vi "dare_verify.vi"(7 "Answer":T1, 8 "Q":T1, 9 "R":T1, 10 "B":T1, 11 "A":T1) -> (0 "Eigenvalues":cdb[](array[numeric]), 1 "ZERO":T1, 3 "Passed":bool)   [LabVIEW 2019]
uses:
  <vilib>/Analysis/Matrix/Datatypes/RealMatrix.ctl
  <vilib>/Analysis/7linalg.llb/Eigenvalue and Vectors Output Option.ctl
  <vilib>/Analysis/7linalg.llb/Real Transpose Matrix.vi
  <vilib>/Analysis/baseanly.llb/Real A x B.vi
  <vilib>/Analysis/Matrix/Numeric/Subtract/Subtract - RM,RM.vi
  <vilib>/Analysis/Matrix/Numeric/Absolute Value/Absolute Value - RM.vi
  <vilib>/Analysis/7linalg.llb/Real Eigenvalues and Vectors.vi
  <vilib>/Analysis/Matrix/Numeric/Add/Add - RM,RM.vi
  <vilib>/Analysis/baseanly.llb/Real Inverse Matrix.vi
  <vilib>/Analysis/NI_AALPro.lvlib
  <vilib>/Analysis/NI_AALBase.lvlib
  <vilib>/Analysis/Matrix/NI_Matrix.lvlib
  <vilib>/Rock Robotics/WPI/ThirdParty/JAS_Junk/TrajLib/Trajectory_Library.lvlib
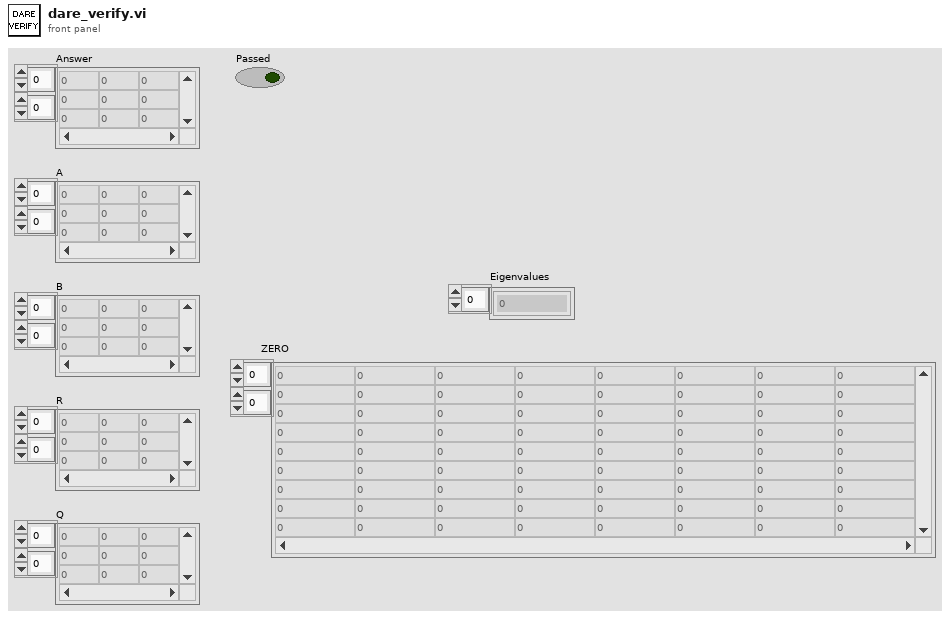
[diagram p1: front panel]
types:
  T1 = typedef "NI_Matrix.lvlib/RealMatrix.ctl" = dbl[][]
  T2 = typedef "NI_AALPro.lvlib/Eigenvalue and Vectors Output Option.ctl" = i32
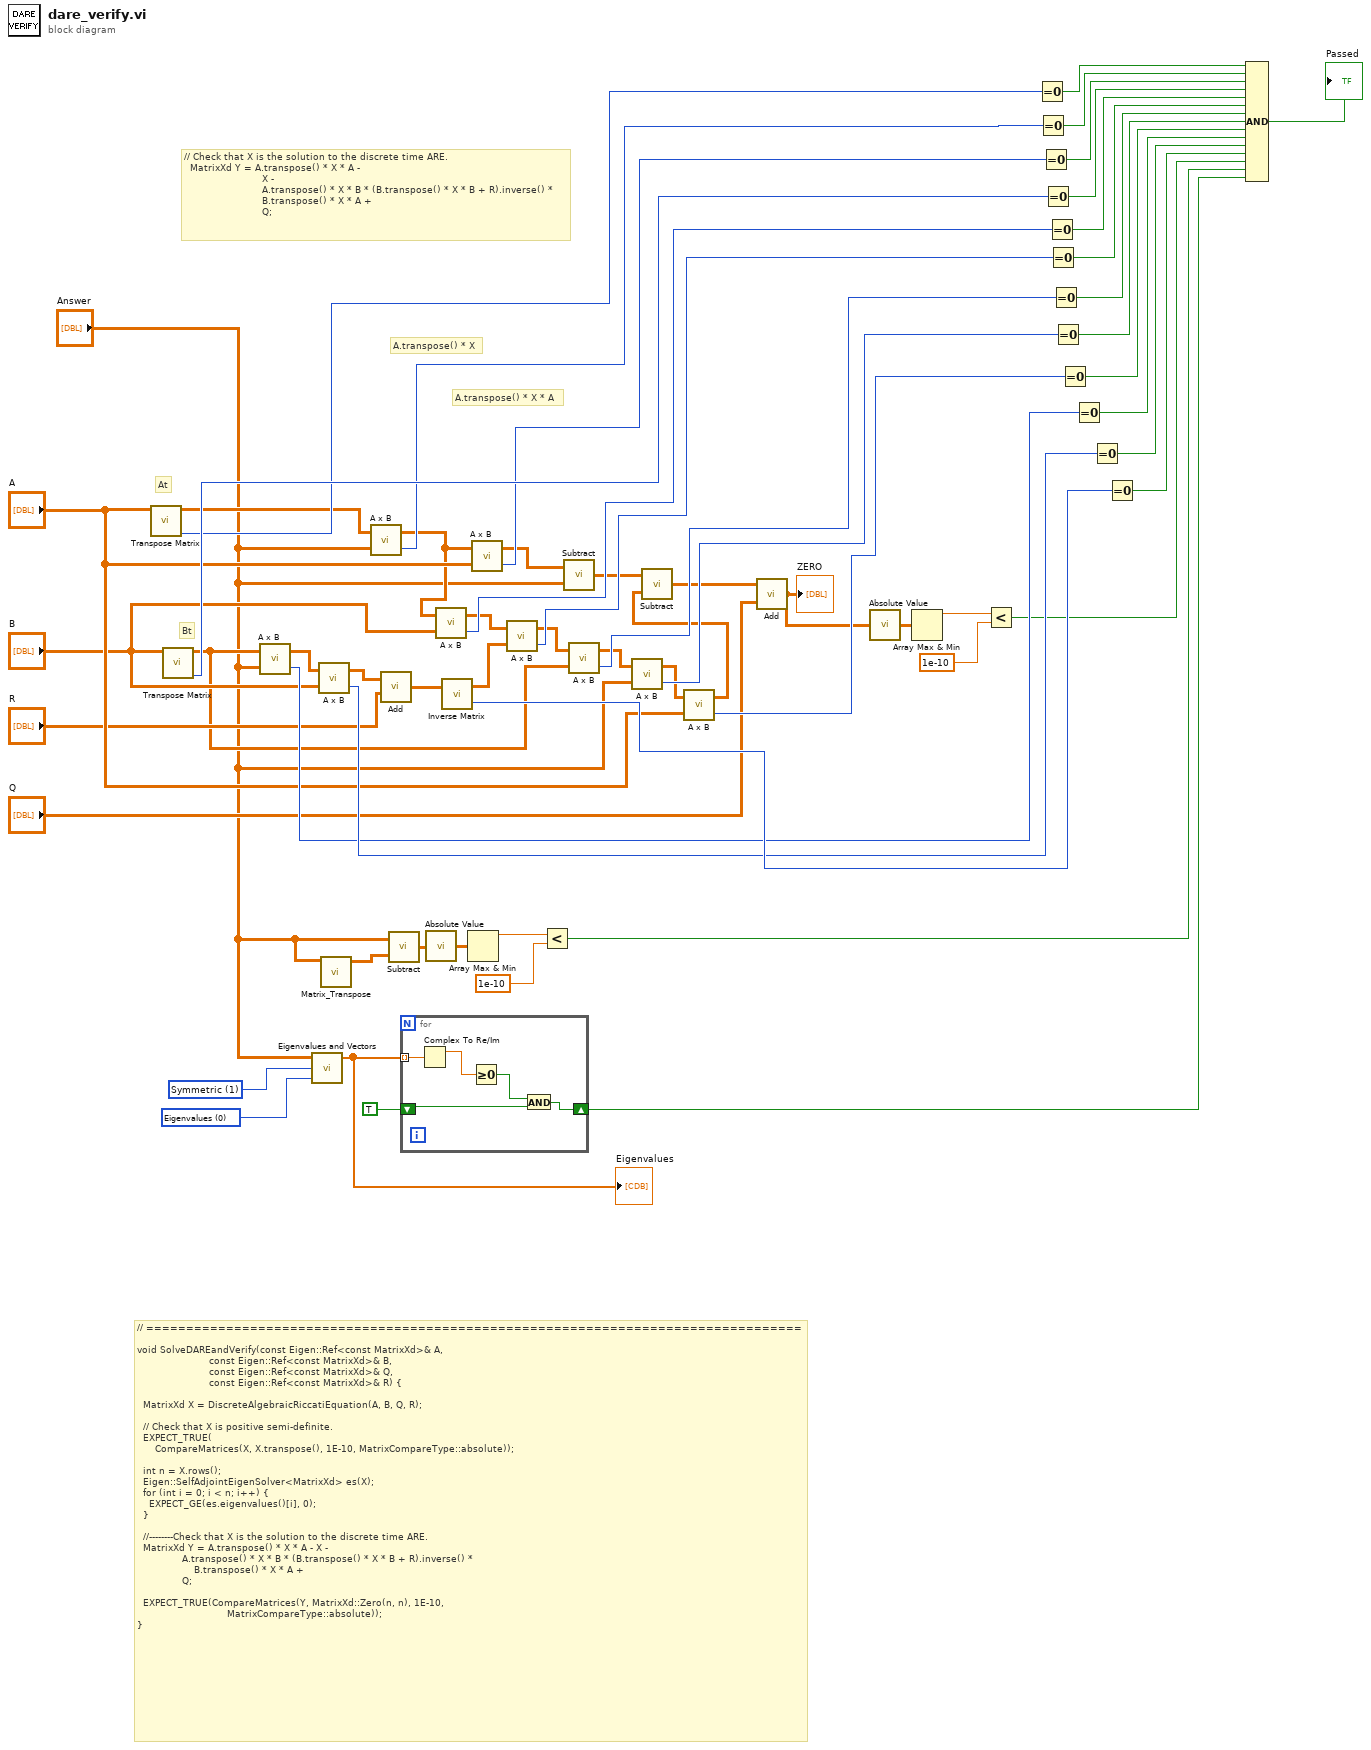
[diagram p0: block diagram]
diagram:
  w4 = T2 0 items=["Eigenvalues", "Eigenvalues & Vectors"] ("output option")
  w5 = 1 items=["General", "Symmetric"] ("matrix type")
  # "// ==================================================================================\n\nvoid SolveDAREandVerify(const Eigen::Ref<const MatrixXd>& A,\n                        const Eigen::Ref<const MatrixXd>& B,\n                        const Eigen::Ref<const MatrixXd>& Q,\n                        const Eigen::Ref<const MatrixXd>& R) {\n\n  MatrixXd X = DiscreteAlgebraicRiccatiEquation(A, B, Q, R);\n\n  // Check that X is positive semi-definite.\n  EXPECT_TRUE(\n      CompareMatrices(X, X.transpose(), 1E-10, MatrixCompareType::absolute));\n\n  int n = X.rows();\n  Eigen::SelfAdjointEigenSolver<MatrixXd> es(X);\n  for (int i = 0; i < n; i++) {\n    EXPECT_GE(es.eigenvalues()[i], 0);\n  }\n\n  //--------Check that X is the solution to the discrete time ARE.\n  MatrixXd Y = A.transpose() * X * A - X -\n               A.transpose() * X * B * (B.transpose() * X * B + R).inverse() *\n                   B.transpose() * X * A +\n               Q;\n\n  EXPECT_TRUE(CompareMatrices(Y, MatrixXd::Zero(n, n), 1E-10,\n                              MatrixCompareType::absolute));\n}"
  # "A.transpose() * X"
  # "A.transpose() * X * A"
  # "Bt"
  # "At"
  # "// Check that X is the solution to the discrete time ARE.\n  MatrixXd Y = A.transpose() * X * A - \n                          X -\n                          A.transpose() * X * B * (B.transpose() * X * B + R).inverse() *\n                          B.transpose() * X * A +\n                          Q;"
  n1 = call-poly <vilib>:"Transpose Matrix.vi"("Input Matrix"="A") -> ("error"=w50:i32, "Matrix Transpose"=w27:T1)  [unwired: 9 in]
  n2 = call-poly <vilib>:"Transpose Matrix.vi"("Input Matrix"="B") -> ("error"=w53:i32, "Matrix Transpose"=w19:T1)  [unwired: 9 in]
  n3 = call-poly <vilib>:"A x B.vi"("B"="Answer", "A"=w19) -> ("error"=w59:i32, "A x B"=w14:T1)
  n4 = call-poly <vilib>:"Eigenvalues and Vectors.vi"("output option"=w4, "matrix type"=w5, "Input Matrix"="Answer") -> ("Eigenvalues"=w3:cdb[])  [unwired: 2 out]
  "Eigenvalues" <- w3
  n5 = call-poly <vilib>:"A x B.vi"("B"="B", "A"=w14) -> ("error"=w60:i32, "A x B"=w15:T1)
  n6 = call <vilib>:"Matrix_Transpose.vi"("input matrix"="Answer") -> ("output matrix"=w12:T1)  [unwired: 10 in]
  n7 = call-poly <vilib>:"A x B.vi"("B"="Answer", "A"=w27) -> ("error"=w51:i32, "A x B"=w25:T1)
  n8 = call-poly <vilib>:"Add.vi"("Real Matrix B"="R", "Real Matrix A"=w15) -> ("A + B"=w16:T1)
  n9 = call-poly <vilib>:"Subtract.vi"("Real Matrix B"=w12, "Real Matrix A"="Answer") -> ("A - B"=w8:T1)
  n10 = for {
    tunnel: w3 -> [w66] mode=indexing
    shift-right: [w62] -> w1
    shift-left: TRUE -> [w63]
    n11 = Complex To Re/Im(x + iy=w66) -> (x=w65:dbl)  [unwired: 1 out]
    n12 = Greater Or Equal To 0?(x=w65) -> (x >= 0?=w64:bool)
    n13 = And(x=w64, y=w63) -> (x .and. y?=w62:bool)
  }
  n14 = call-poly <vilib>:"Absolute Value.vi"("Real Matrix A"=w8) -> ("|A|"=w9:T1)
  n15 = call-poly <vilib>:"A x B.vi"("B"="B", "A"=w25) -> ("error"=w54:i32, "A x B"=w26:T1)
  n16 = call-poly <vilib>:"Inverse Matrix.vi"("Input Matrix"=w16) -> ("error"=w61:i32, "Inverse Matrix"=w17:T1)  [unwired: 1 in]
  n17 = Array Max & Min(array=w9) -> (max value=w10:dbl)  [unwired: 3 out]
  n18 = call-poly <vilib>:"A x B.vi"("B"="A", "A"=w25) -> ("error"=w52:i32, "A x B"=w13:T1)
  n19 = call-poly <vilib>:"A x B.vi"("B"=w17, "A"=w26) -> ("error"=w55:i32, "A x B"=w18:T1)
  n20 = Less?(x=w10, y=1e-10) -> (x < y?=w7:bool)
  n21 = call-poly <vilib>:"Subtract.vi"("Real Matrix B"="Answer", "Real Matrix A"=w13) -> ("A - B"=w22:T1)
  n22 = call-poly <vilib>:"A x B.vi"("B"=w19, "A"=w18) -> ("error"=w56:i32, "A x B"=w20:T1)
  n23 = call-poly <vilib>:"A x B.vi"("B"="Answer", "A"=w20) -> ("error"=w57:i32, "A x B"=w21:T1)
  n24 = call-poly <vilib>:"A x B.vi"("B"="A", "A"=w21) -> ("error"=w58:i32, "A x B"=w23:T1)
  n25 = call-poly <vilib>:"Subtract.vi"("Real Matrix B"=w23, "Real Matrix A"=w22) -> ("A - B"=w24:T1)
  n26 = call-poly <vilib>:"Add.vi"("Real Matrix B"="Q", "Real Matrix A"=w24) -> ("A + B"=w49:T1)
  "ZERO" <- w49
  n27 = call-poly <vilib>:"Absolute Value.vi"("Real Matrix A"=w49) -> ("|A|"=w45:T1)
  n28 = Array Max & Min(array=w45) -> (max value=w46:dbl)  [unwired: 3 out]
  n29 = Less?(x=w46, y=1e-10) -> (x < y?=w48:bool)
  n30 = Equal To 0?(x=w50) -> (x = 0?=w33:bool)
  n31 = Equal To 0?(x=w51) -> (x = 0?=w34:bool)
  n32 = Equal To 0?(x=w52) -> (x = 0?=w35:bool)
  n33 = Equal To 0?(x=w53) -> (x = 0?=w36:bool)
  n34 = Equal To 0?(x=w54) -> (x = 0?=w37:bool)
  n35 = Equal To 0?(x=w55) -> (x = 0?=w38:bool)
  n36 = Equal To 0?(x=w56) -> (x = 0?=w39:bool)
  n37 = Equal To 0?(x=w57) -> (x = 0?=w40:bool)
  n38 = Equal To 0?(x=w58) -> (x = 0?=w41:bool)
  n39 = Equal To 0?(x=w59) -> (x = 0?=w42:bool)
  n40 = Equal To 0?(x=w60) -> (x = 0?=w43:bool)
  n41 = Equal To 0?(x=w61) -> (x = 0?=w44:bool)
  n42 = Compound Arithmetic op=AND(w33, w34, w35, w36, w37, w38, w39, w40, w41, w42, w43, w44, w48, w7, w1) -> (→"Passed":bool)
